vi "GEOM_FPA2DetROI.vi"(7 "ROIcoords":T4={"xstart"=1, "ystart"=1, "xsize"=1, "ysize"=1}, 9 "clean first?":bool, 10 "amplifiers":T1[](array[typedef]) {"fliped" items=["none", "horizontal", "vertical"]; "type" items=["LL", "LR", "UL", "UR"]}, 11 "CorrectionType":T5) -> (2 "amplifiers out":T1[](array[typedef]) {"fliped" items=["none", "horizontal", "vertical"]; "type" items=["LL", "LR", "UL", "UR"]})   [LabVIEW 2016]
doc: "This VI transform a global ROI (FPA ROI) to individual ROIs per amplifier. This means that the input is the amplifier list and the global ROI , and the output are the amplifier list with the original ROI requsted FOR THAT amplifier, and the ROI corrected for that amplifier. The corrections to apply will depend on the capabilities of the electronics (can it send just the selected area, all or always all the columns?, for example)"
uses:
  GEOM_Amplifier.ctl
  GEOM_AmpType.ctl
  GEOM_ROI.ctl
  GEOM_Coords.ctl
  GEOM_ROICorrection.ctl
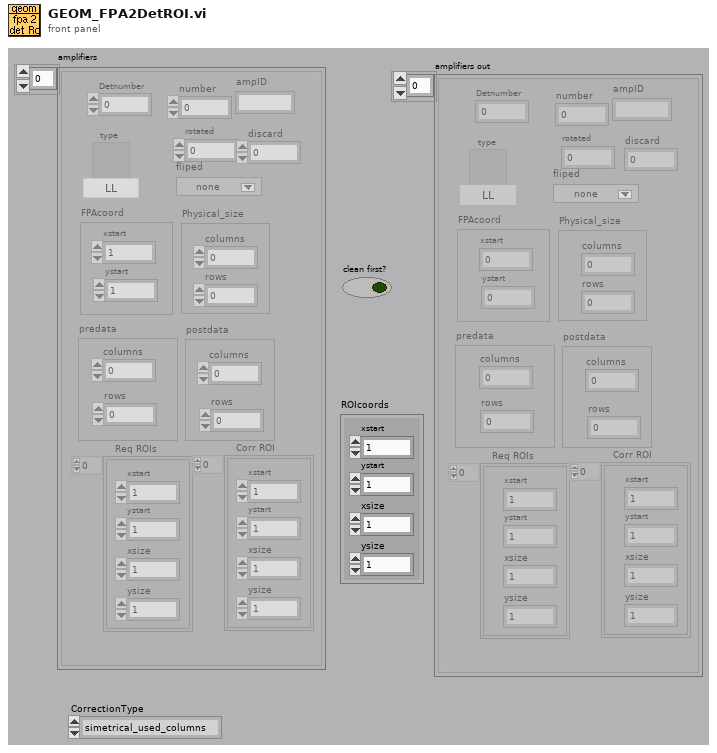
[diagram p1: front panel]
types:
  T1 = typedef "GEOM_Amplifier.ctl" = cluster{"number":i32, "type":T2, "rotated":i16, "fliped":u16, "FPAcoord":cluster{"xstart":i32, "ystart":i32}, "Physical_size":cluster{"columns":i32, "rows":i32}, "predata":cluster{"columns":i32, "rows":i32}, "postdata":cluster{"columns":i32, "rows":i32}, "Req ROIs":T3, "Corr ROI":T3, "Detnumber":i32, "ampID":string, "discard":i32}
  T2 = typedef "GEOM_AmpType.ctl" = u16
  T3 = typedef "GEOM_ROI.ctl" = T4[]
  T4 = typedef "GEOM_Coords.ctl" = cluster{"xstart":u32, "ystart":u32, "xsize":u32, "ysize":u32}
  T5 = typedef "GEOM_ROICorrection.ctl" = enum16{"simetrical_used_columns", "simetrical_all_columns"}
  T6 = cluster{"xstart":i32, "ystart":i32, "columns":i32, "rows":i32}
  T7 = cluster{"xstart":i32, "ystart":i32, "xend":i32, "yend":i32}
  T8 = cluster{"xrs":i32, "yrs":i32, "xre":i32, "yre":i32}
  T9 = cluster{"xstart":i32, "ystart":i32, "xend":i32, "yend":i32}[]
  T10 = cluster{"xstart":i32, "ystart":i32, "xsize":i32, "ysize":i32}
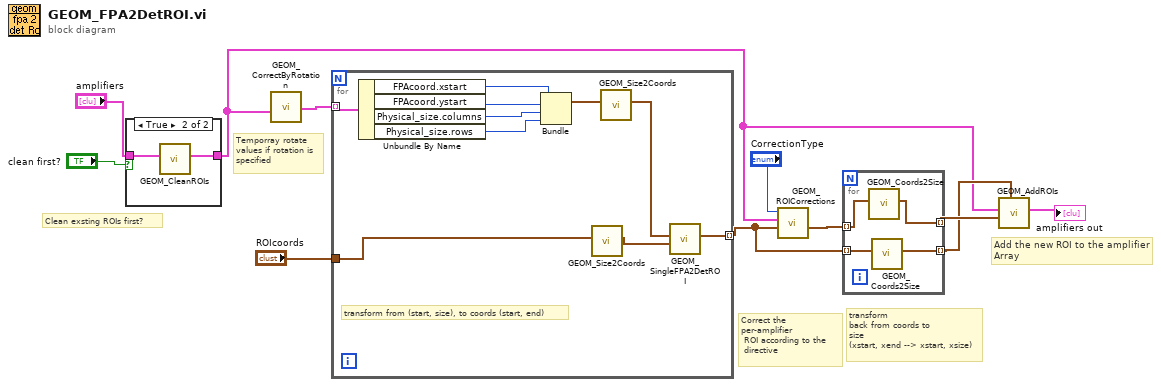
[diagram p0: block diagram]
diagram:
  # "Temporray rotate\nvalues if rotation is\nspecified"
  # "transform\nback from coords to\nsize \n(xstart, xend --> xstart, xsize)"
  # "Add the new ROI to the amplifier \nArray"
  # "Correct the \nper-amplifier\n ROI according to the\n directive"
  # "Clean exsting ROIs first?"
  n1 = case shown="True" "clean first?" {
    tunnel: "amplifiers" -> [w12 w14]
    tunnel: [w12 w13] -> w2
    frame False {
    }
    frame True {
      n2 = call "GEOM_CleanROIs.vi"("amplifiers in"=w14) -> ("amplifiers out"=w13:T1[])  [unwired: 1 in, 9 out]
    }
  }
  n3 = call "GEOM_CorrectByRotation.vi"("Amplifiers"=w2) -> ("rotated amps"=w1:T1[])  [unwired: 1 in, 9 out]
  n4 = for {
    tunnel: w1 -> [w24] mode=indexing
    tunnel: "ROIcoords" -> [w17]
    tunnel: [w23] -> w4 mode=indexing
    # "transform from (start, size), to coords (start, end)"
    n5 = Unbundle By Name(w24) -> ("FPAcoord.xstart"=w22:i32, "FPAcoord.ystart"=w21:i32, "Physical_size.columns"=w20:i32, "Physical_size.rows"=w19:i32)
    n6 = Bundle("xstart"=w22, "ystart"=w21, "columns"=w20, "rows"=w19) -> (w18:T6)  [unwired: 1 out]
    n7 = call "GEOM_Size2Coords.vi"("Size"=w17) -> ("Coords"=w16:T7)  [unwired: 10 out]
    n8 = call "GEOM_Size2Coords.vi"("Size"=w18) -> ("Coords"=w15:T7)  [unwired: 10 out]
    n9 = call "GEOM_SingleFPA2DetROI.vi"("FPAROIcoords"=w16, "FPAampcoords"=w15) -> ("ROI det coords"=w23:T8)  [unwired: 9 out]
  }
  n10 = call "GEOM_ROICorrections.vi"("ROIS"=w4, "amplifiers"=w2, "CorrectionType"="CorrectionType") -> ("Corrected ROIs"=w8:T9)  [unwired: 8 out]
  n11 = for {
    tunnel: w8 -> [w28] mode=indexing
    tunnel: [w27] -> w7 mode=indexing
    tunnel: w4 -> [w26] mode=indexing
    tunnel: [w25] -> w3 mode=indexing
    n12 = call "GEOM_Coords2Size.vi"("Coords"=w28) -> ("Size"=w27:T10)  [unwired: 10 out]
    n13 = call "GEOM_Coords2Size.vi"("Coords"=w26) -> ("Size"=w25:T10)  [unwired: 10 out]
  }
  n14 = call "GEOM_AddROIs.vi"("Requested ROIs"=w3, "Corrrected ROIs"=w7, "amplifiers in"=w2) -> ("amplifiers out"=→"amplifiers out":T1[])  [unwired: 8 out]
